vi "problem3-Client.vi"() -> ()   [LabVIEW 2017]
panel:
  out "x*y":cluster{i32}
  out "x+y":cluster{i32}
  out "error out":errorcluster
  in  "stop":bool
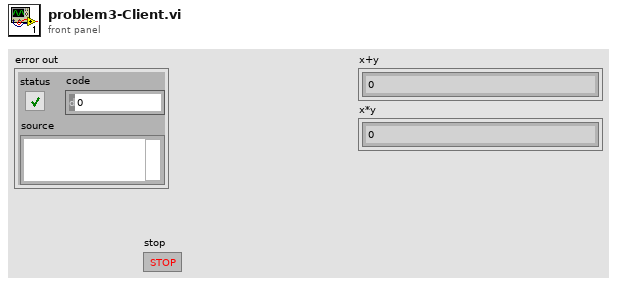
[diagram p1: front panel]
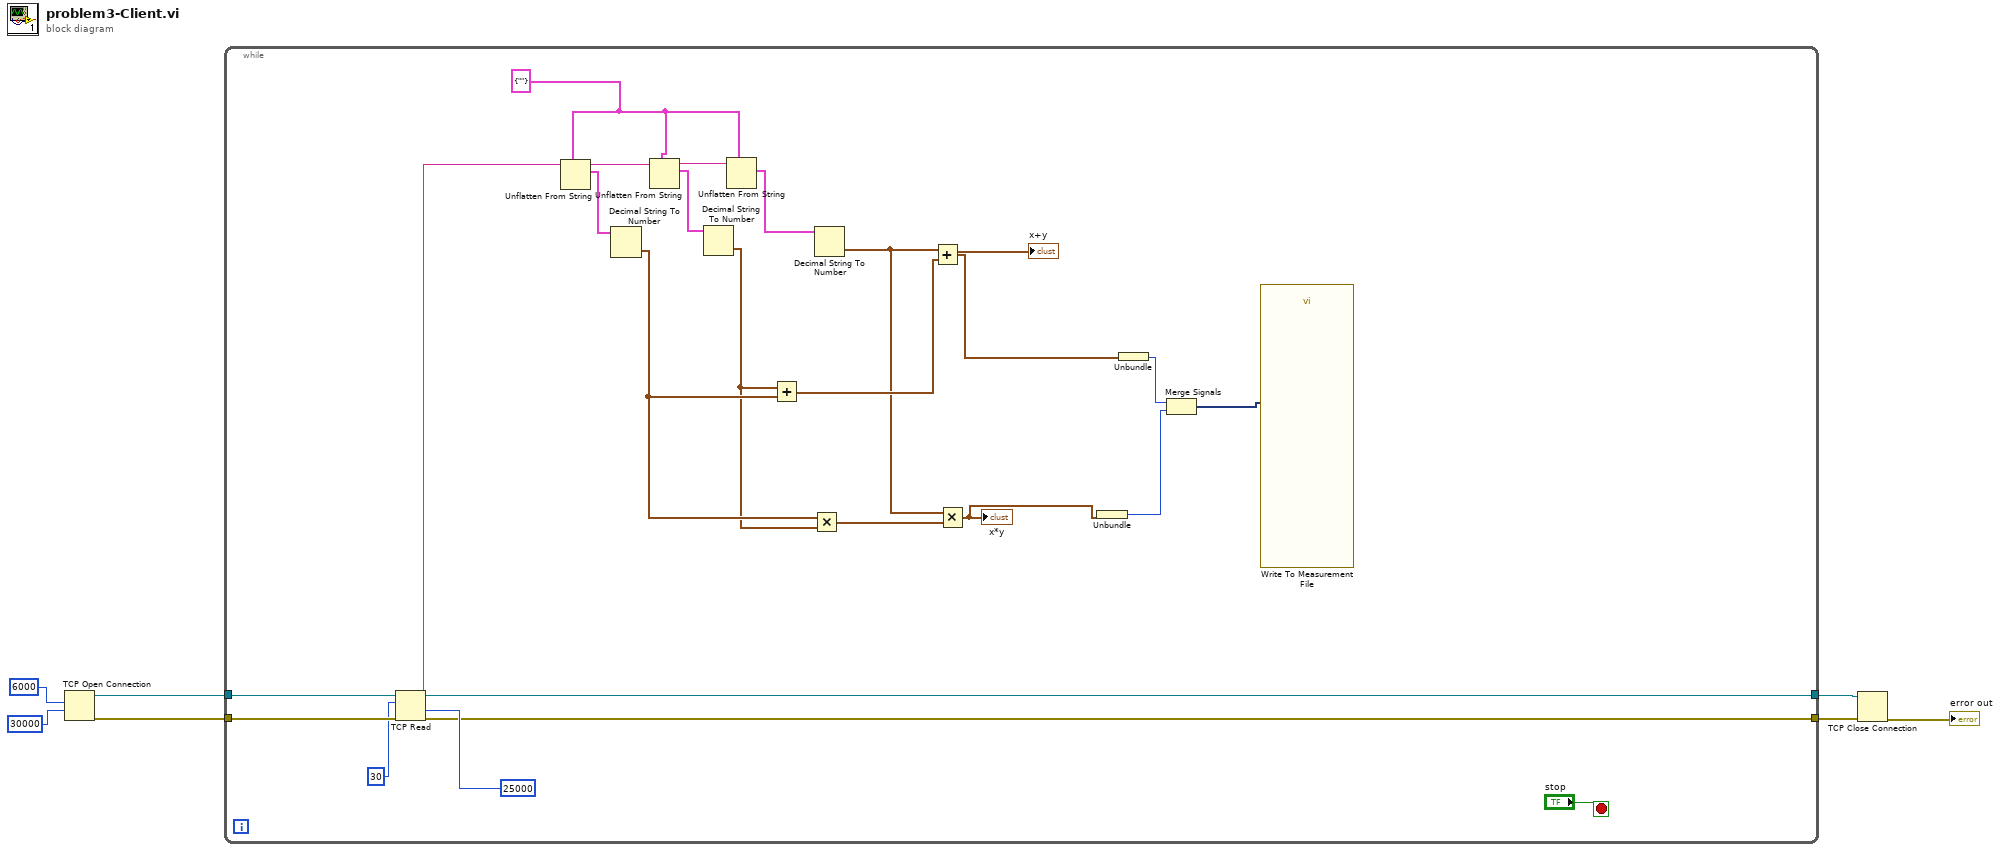
[diagram p0: block diagram]
diagram:
  n1 = TCP Open Connection(remote port or service name=u16 6000, timeout ms (60000)=30000) -> (connection ID=w7:refnum<k5>, error out=w6:errorcluster)  [unwired: 3 in]
  n2 = while {
    tunnel: w7 -> [w30]
    tunnel: w6 -> [w29]
    tunnel: [w14] -> w2
    tunnel: [w13] -> w1
    stop <- "stop" stop-if-true
    w24 = cluster{string} {""} ("type")
    n3 = TCP Read(connection ID=w30, bytes to read=30, error in (no error)=w29, 9:25000 ("timeout ms (25000)")) -> (connection ID out=w14:refnum<k5>, data out=w27:string, error out=w13:errorcluster)  [unwired: 1 in]
    n4 = Unflatten From String(type=w24, binary string=w27) -> (rest of the binary string=w26:string, value=w23:cluster{string})  [unwired: 3 in, 1 out]
    n5 = Decimal String To Number(string=w23) -> (number=w19:cluster{i32})  [unwired: 2 in, 1 out]
    n6 = Unflatten From String(type=w24, binary string=w26) -> (rest of the binary string=w25:string, value=w22:cluster{string})  [unwired: 3 in, 1 out]
    n7 = Decimal String To Number(string=w22) -> (number=w18:cluster{i32})  [unwired: 2 in, 1 out]
    n8 = Unflatten From String(type=w24, binary string=w25) -> (value=w21:cluster{string})  [unwired: 3 in, 2 out]
    n9 = Add(x=w18, y=w19) -> (x+y=w20:cluster{i32})
    n10 = Multiply(x=w19, y=w18) -> (x*y=w16:cluster{i32})
    n11 = Decimal String To Number(string=w21) -> (number=w17:cluster{i32})  [unwired: 2 in, 1 out]
    n12 = Add(x=w17, y=w20) -> (x+y=w12:cluster{i32})
    "x+y" <- w12
    n13 = Multiply(x=w17, y=w16) -> (x*y=w10:cluster{i32})
    "x*y" <- w10
    n14 = Unbundle(w10) -> (w8:i32)
    n15 = Unbundle(w12) -> (w11:i32)
    n16 = Merge Signals(w11, w8) -> (w9:dynamicdata)
    n17 = call "Write To Measurement File"("Signals"=w9) -> ()  [unwired: 16 in, 3 out]
  }
  n18 = TCP Close Connection(connection ID=w2, error in (no error)=w1) -> (error out=→"error out":errorcluster)  [unwired: 1 in, 1 out]
